vi "write slope info FROM clusters.vi"(2 "Output Slopes Cluster in":T1, 3 "Input Variables and Slopes in":T2 {"Height of Sample Box" format="%.2f"; "Reservoir Pressure" format="%.2f"; "Flow Offset" format="%.2f"; "String Pot Offset" format="%.2f"; "Aux 3 Offset" format="%.2f"; "Aux 2 Offset" format="%.2f"; "Aux 1 Offset" format="%.2f"; "Aux 3 Slope" format="%.2f"; "Aux 2 Slope" format="%.2f"; "Aux 1 Slope" format="%.2f"; "Up Hole  Pressure Offset" format="%.2f"; "DH Pressure Offset" format="%.2f"; "DH Pressure Trans Slope" format="%.2f"; "Atmospheric Pressure" format="%.2f"; "Depth to Water Table" format="%.2f"; "Up Hole Pressure Slope" format="%.2f"; "Flow Slope" format="%.2f"; "String Pot Slope" format="%.2f"; "Total Volume" format="%.2f"}) -> (0 "DHT_Pressure_ Offset":dbl, 1 "DHT_Pressure Slope":dbl, 4 "Input Variables and Slopes out":T2 {"Height of Sample Box" format="%.2f"; "Reservoir Pressure" format="%.2f"; "Flow Offset" format="%.2f"; "String Pot Offset" format="%.2f"; "Aux 3 Offset" format="%.2f"; "Aux 2 Offset" format="%.2f"; "Aux 1 Offset" format="%.2f"; "Aux 3 Slope" format="%.2f"; "Aux 2 Slope" format="%.2f"; "Aux 1 Slope" format="%.2f"; "Up Hole  Pressure Offset" format="%.2f"; "DH Pressure Offset" format="%.2f"; "DH Pressure Trans Slope" format="%.2f"; "Atmospheric Pressure" format="%.2f"; "Depth to Water Table" format="%.2f"; "Up Hole Pressure Slope" format="%.2f"; "Flow Slope" format="%.2f"; "String Pot Slope" format="%.2f"; "Total Volume" format="%.2f"}, 5 "Aux1_Slope out":dbl, 6 "Output Slopes Cluster out":T1, 7 "pressure_slope_Out":dbl, 9 "Aux2_Slope In":dbl, 12 "Aux3_ Slope Out":dbl, 13 "string_pot_slope_Out":dbl, 14 "flow_slope_IN":dbl)   [LabVIEW 2016]
uses:
  KPRO_2016 subvis/Control 2.ctl
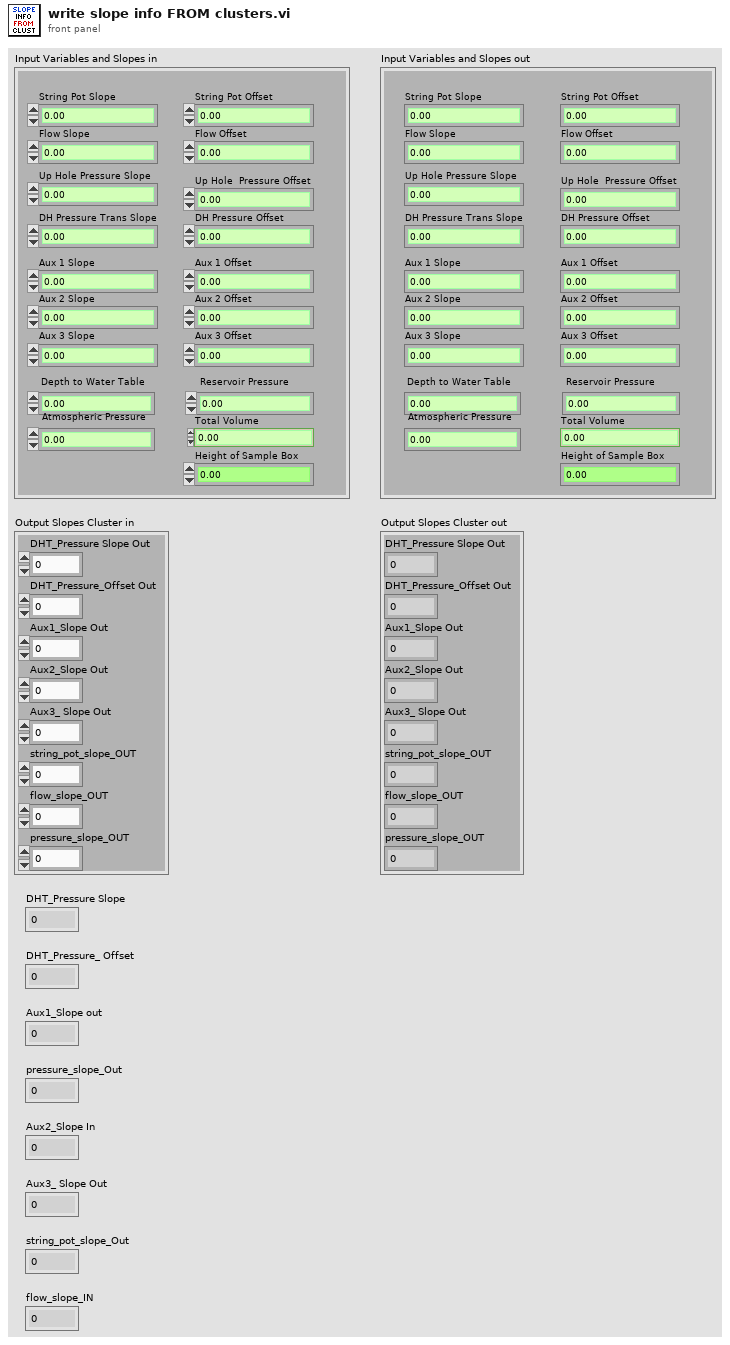
[diagram p1: front panel]
types:
  T1 = cluster{"DHT_Pressure Slope Out":dbl, "DHT_Pressure_Offset Out":dbl, "Aux1_Slope Out":dbl, "Aux2_Slope Out":dbl, "Aux3_ Slope Out":dbl, "string_pot_slope_OUT":dbl, "flow_slope_OUT":dbl, "pressure_slope_OUT":dbl}
  T2 = typedef "Control 2.ctl" = cluster{"Total Volume":dbl, "String Pot Slope":dbl, "Flow Slope":dbl, "Up Hole Pressure Slope":dbl, "Depth to Water Table":dbl, "Atmospheric Pressure":dbl, "DH Pressure Trans Slope":dbl, "DH Pressure Offset":dbl, "Up Hole  Pressure Offset":dbl, "Aux 1 Slope":dbl, "Aux 2 Slope":dbl, "Aux 3 Slope":dbl, "Aux 1 Offset":dbl, "Aux 2 Offset":dbl, "Aux 3 Offset":dbl, "String Pot Offset":dbl, "Flow Offset":dbl, "Reservoir Pressure":dbl, "Height of Sample Box":dbl}
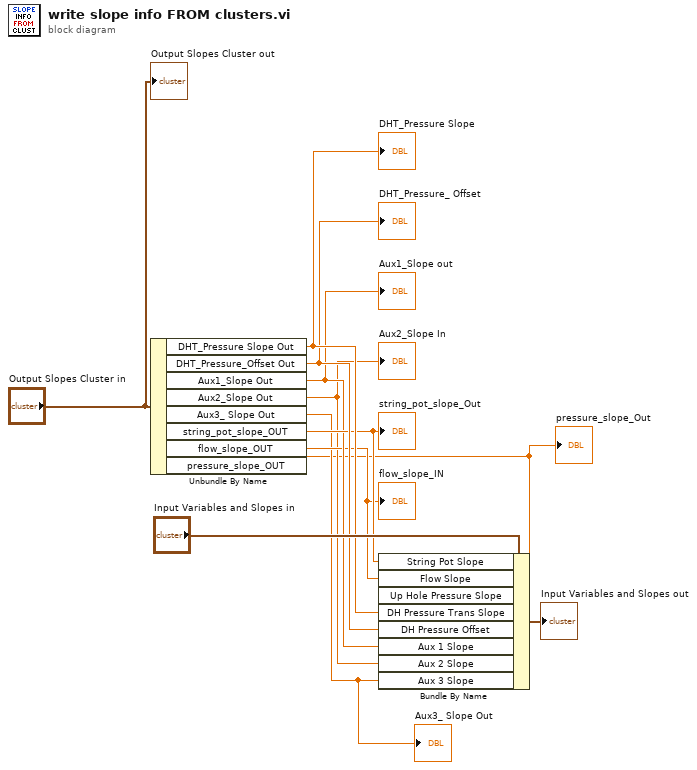
[diagram p0: block diagram]
diagram:
  n1 = Unbundle By Name("Output Slopes Cluster in") -> ("DHT_Pressure Slope Out"=w8:dbl, "DHT_Pressure_Offset Out"=w7:dbl, "Aux1_Slope Out"=w5:dbl, "Aux2_Slope Out"=w3:dbl, "Aux3_ Slope Out"=w2:dbl, "string_pot_slope_OUT"=w6:dbl, "flow_slope_OUT"=w4:dbl, "pressure_slope_OUT"=w1:dbl)
  "Aux3_ Slope Out" <- w2
  "Aux2_Slope In" <- w3
  "Aux1_Slope out" <- w5
  "DHT_Pressure_ Offset" <- w7
  "DHT_Pressure Slope" <- w8
  "pressure_slope_Out" <- w1
  "flow_slope_IN" <- w4
  "string_pot_slope_Out" <- w6
  n2 = Bundle By Name(cluster="Input Variables and Slopes in", "String Pot Slope"=w6, "Flow Slope"=w4, "Up Hole Pressure Slope"=w1, "DH Pressure Trans Slope"=w8, "DH Pressure Offset"=w7, "Aux 1 Slope"=w5, "Aux 2 Slope"=w3, "Aux 3 Slope"=w2) -> (→"Input Variables and Slopes out":T2)
  "Output Slopes Cluster out" <- "Output Slopes Cluster in"
